vi "Update.vi"(8 "Error In":errorcluster, 10 "Option String":string, 11 "Tree Data In":refnum<class "Tree Data.lvclass">) -> (0 "Error Out":errorcluster, 3 "Tree Data Out":refnum<class "Tree Data.lvclass">)   [LabVIEW 2020, in "NI_VIAnCFGDataStructure.lvlib" / "Tree Data.lvclass"]
doc: "This is an abstract method defining an interface for Tree Data Update functionality, invoked in the Tree API with Update method. Override it in child classes."
uses:
  <vilib>/addons/analyzer/VIAnCFGDataStructure/Tree Data/Tree Data.lvclass
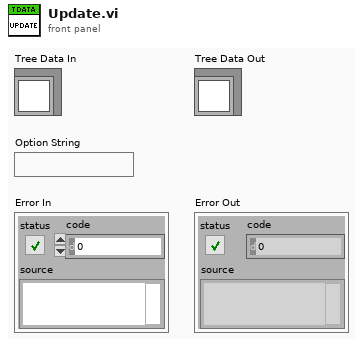
[diagram p1: front panel]
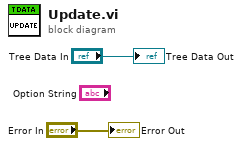
[diagram p0: block diagram]
diagram:
  "Tree Data Out" <- "Tree Data In"
  "Error Out" <- "Error In"
